vi "Clock Cross Produce.vi"(0 "register instruction":T1, 2 "resources":T2) -> (14 "ready for input":bool)   [LabVIEW 2020]
doc: "Takes register instructions from the register bus process and enqueues them to be consumed in the other clock domain.\n\n<B>Input Parameters</B>\n\n<B>resources</B> contains references to the clock crossing FIFOs.\n\n<B>register instruction</B> is the register bus instruction to enqueue.\n\n<B>Output Parameters</B>\n\n<B>ready for input</B> is a flow control signal that indicates whether this VI is ready to accept a new instruction."
uses:
  Clock Cross Resources.ctl
  <instrlib>/_niInstr/Register Bus/v1/FPGA/Public/Register Instruction.ctl
  <vilib>/rvi/DataTransferAndStorage/Container/Common/niFpgaContainerExecOnDevCompGetState.vi
  <vilib>/rvi/Emulation/niFpgaEmulationIsFPGAContextNoSignature.vi
  <vilib>/rvi/Emulation/niFpgaSctlEmulationGetInTimedLoop.vi
  <vilib>/rvi/errors/niFpgaSetErrorForExecOnDevCompSimple.vi
  <vilib>/rvi/eio/common/nirviEmuReportErrorAndStop.vi
  <vilib>/rvi/DataTransferAndStorage/Container/Common/niFpgaContainerGetUniqueNameForEmu.vi
  <vilib>/rvi/FIFO/Fifo_Resource/nirvififoEmulationSetSize.vi
  <vilib>/rvi/FIFO/Fifo_Resource/nirviFifoEmulationQueueMgr.vi
  <instcachedir>/0/nirviFifoEmulationQueueMgr_E5CAEC123FF24DC58D834DCA3CDAA9B5.lvgen/nirviFifoEmulationQueueMgr_E5CAEC123FF24DC58D834DCA3CDAA9B5_007.vi
  <vilib>/rvi/FIFO/Fifo_Resource/nirvififoEmulationDetermineInputValidOut.vi
  <vilib>/rvi/FIFO/Fifo_Resource/nirvififoEmulationCreateLock.vi
  <vilib>/rvi/Emulation/niFpgaProcessEmulError.vi
  <vilib>/rvi/FIFO/Fifo_Resource/nirvififoEmulationObtainLock.vi
  <vilib>/rvi/FIFO/Fifo_Resource/nirvififoEmulationReleaseLock.vi
  <vilib>/rvi/occurrence/nirviWaitOnOccurrenceBase.vi
  <vilib>/rvi/errors/nirviReportUnexpectedCaseInternalError.vi
  <vilib>/rvi/errors/nirviReportUnexpectedCaseInternalError (U32).vi
  <vilib>/Utility/error.llb/Clear Errors.vi
  <vilib>/rvi/interface/RandomDataEmulation/niFpgaRandomDataHandleErrors.vi
  <vilib>/rvi/eio/common/nirviEmuTemplateMethod_errors.vi
  <vilib>/rvi/DataTransferAndStorage/Container/XNode/niFpgaContainer.xnode
  <vilib>/rvi/FIFO/Fifo_Resource/niFpgaFifoEmulationRefIn.vi
  <vilib>/eio/EIONode/EIONode.xnode
  <instrlib>/_niInstr/Register Bus/v1/FPGA/niInstr Register Bus v1 FPGA.lvlib
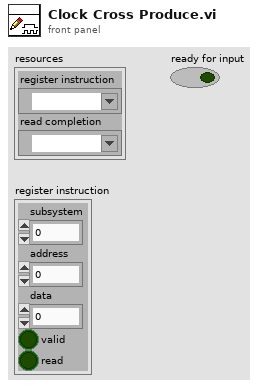
[diagram p1: front panel]
types:
  T1 = typedef "niInstr Register Bus v1 FPGA.lvlib/Register Instruction.ctl" = cluster{"subsystem":u8, "address":u16, "data":u32, "valid":bool, "read":bool}
  T2 = typedef "Clock Cross Resources.ctl" = cluster{"register instruction":refnum<k21>, "read completion":refnum<k21>}
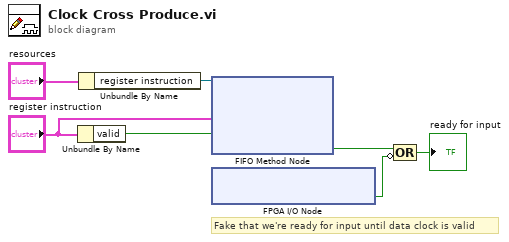
[diagram p0: block diagram]
diagram:
  # "Fake that we're ready for input until data clock is valid"
  n1 = Unbundle By Name("register instruction") -> ("valid"=w4:bool)
  n2 = Unbundle By Name("resources") -> ("register instruction"=w6:refnum<k21>)
  n3 = xnode ("FIFO Method Node")("Element"="register instruction", "Input Valid"=w4, "FIFO In"=w6) -> ("Ready for Input"=w3:bool)  [unwired: 1 out]
  n4 = xnode "FPGA I/O Node"() -> ("Data Clock PLL Locked"=w1:bool)  [unwired: 1 in, 1 out]
  n5 = Compound Arithmetic op=OR(w3, invert w1) -> (→"ready for input":bool)
